vi "error.vi"(11 "error in (no error)":errorcluster) -> ()   [LabVIEW 2018]
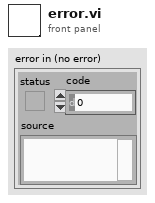
[diagram p1: front panel]
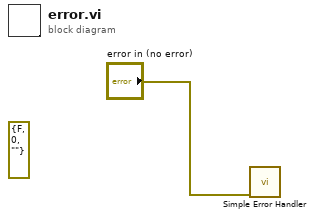
[diagram p0: block diagram]
diagram:
  (unwired) errorcluster {"status"=FALSE, "code"=0, "source"=""} ("error in (no error)")
  n1 = call <vilib>:"Simple Error Handler.vi"("error in (no error)"="error in (no error)") -> ()  [unwired: 4 in, 5 out]
